vi "Convert Units.vi"(1 "Units for Duration Under Test":u8, 2 "Nominal Freq (fnom) Hz":dbl format="%.2f") -> (0 "value":dbl format="%.2f")   [LabVIEW 2021]
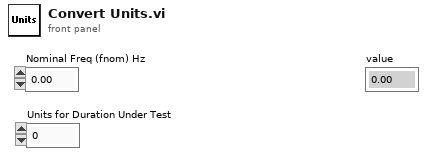
[diagram p1: front panel]
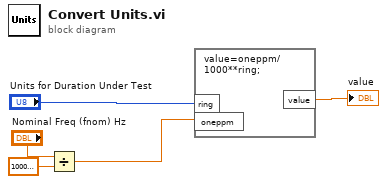
[diagram p0: block diagram]
diagram:
  n1 = Divide(x="Nominal Freq (fnom) Hz", y=1000000.0) -> (x/y=w1:dbl)
  n2 = formula code="value=oneppm/1000**ring;"("ring"="Units for Duration Under Test", "oneppm"=w1) -> ("value"=→"value":dbl)
